vi "Get Communication Line.vi"(8 "error in (no error)":errorcluster, 10 "Excitation":T1=enum."Cy3 (532 nm)", 11 "Laser Quantum in":refnum<class "Laser Quantum.lvclass">) -> (0 "error out":errorcluster, 2 "Serial Port":refnum<visa-resource-name>, 3 "Laser Quantum out":refnum<class "Laser Quantum.lvclass">)   [LabVIEW 2015, in "Laser Quantum.lvlib" / "Laser Quantum.lvclass"]
uses:
  Laser Quantum.lvclass
  Resources/Type Defs/Excitation.ctl
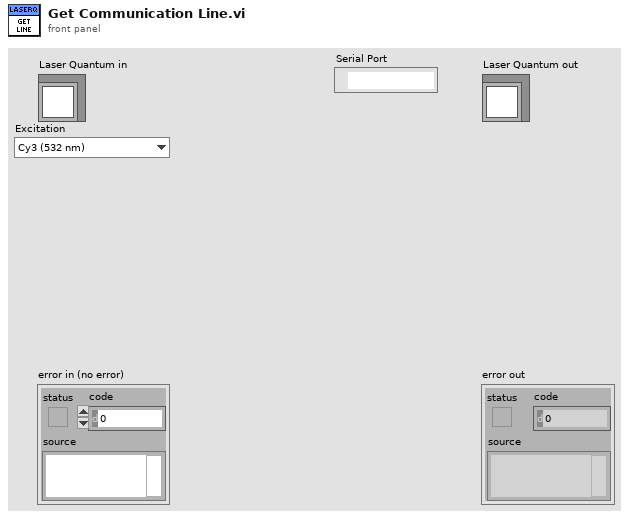
[diagram p1: front panel]
types:
  T1 = typedef "Excitation.ctl" = enum16{"Cy2 (473 nm)", "Cy3 (532 nm)", "Cy5 (639 nm)", "Cy7 (730 nm)"}
  T2 = typedef "Laser Configuration.ctl" = cluster{"Excitation":T1, "Serial Port":refnum<visa-resource-name>}
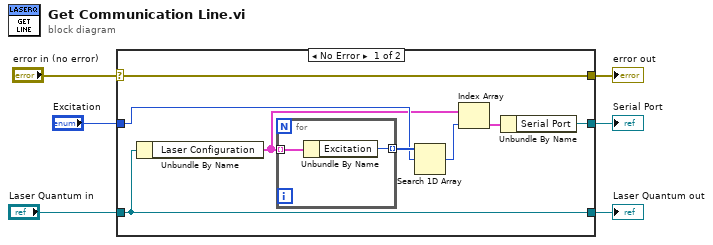
[diagram p0: block diagram]
diagram:
  n1 = case shown="No Error" "error in (no error)" {
    selector: "error in (no error)" -> [w14 w18]
    tunnel: [w14 w18] -> w3
    tunnel: [w9 w17] -> w2
    tunnel: "Laser Quantum in" -> [w9 w17]
    tunnel: "Excitation" -> [w12 _]
    tunnel: [w11 _] -> w1
    frame No Error {
      n2 = Unbundle By Name(w9) -> ("Laser Configuration"=w8:T2[])
      n3 = for {
        tunnel: w8 -> [w16] mode=indexing
        tunnel: [w15] -> w13 mode=indexing
        n4 = Unbundle By Name(w16) -> ("Excitation"=w15:T1)
      }
      n5 = Search 1D Array(1D array=w13, element=w12) -> (index of element=w10:i32)  [unwired: 1 in]
      n6 = Index Array(array=w8, index=w10) -> (element=w7:T2)
      n7 = Unbundle By Name(w7) -> ("Serial Port"=w11:refnum<visa-resource-name>)
    }
    frame Error {
    }
  }
  "error out" <- w3
  "Laser Quantum out" <- w2
  "Serial Port" <- w1
